vi "读取二维数组并转换到簇_new.vi"() -> (11 "Port 0":T1)   [LabVIEW 2021]
uses:
  <vilib>/Utility/file.llb/Read Delimited Spreadsheet (DBL).vi
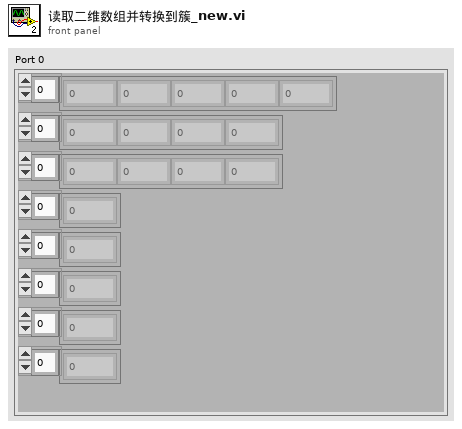
[diagram p1: front panel]
types:
  T1 = cluster{dbl[], dbl[], dbl[], dbl[], dbl[], dbl[], dbl[], dbl[]}
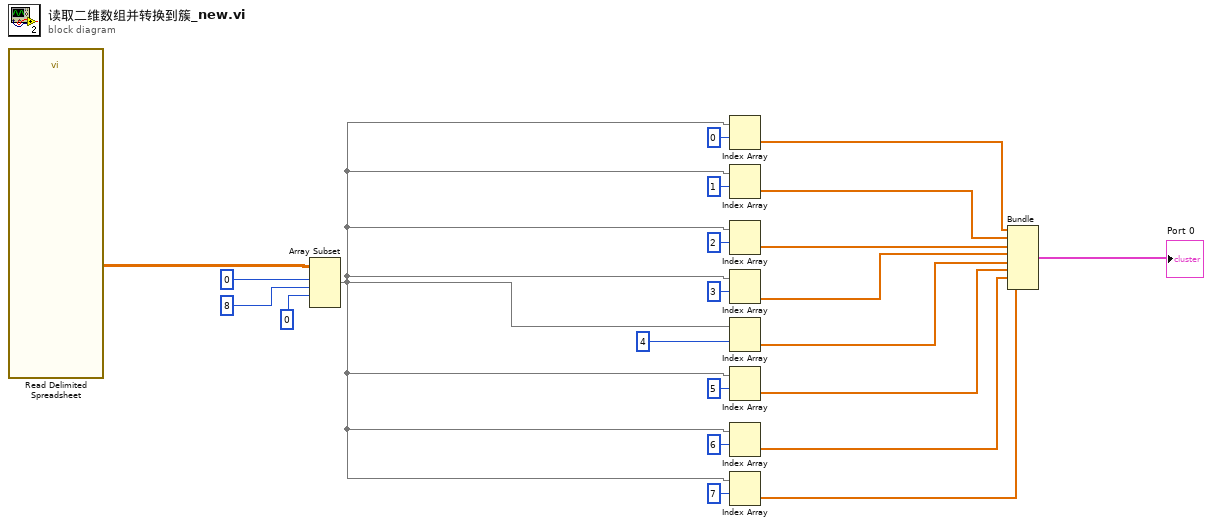
[diagram p0: block diagram]
diagram:
  n1 = call-poly <vilib>:"Read Delimited Spreadsheet.vi"() -> ("all rows"=w1:dbl[][])  [unwired: 10 in, 5 out]
  n2 = Array Subset(array=w1, index (row)=0 ("index"), length (row)=8 ("length"), index (col)=0 ("index")) -> (w12:dbl[][])  [unwired: 1 in]
  n3 = Index Array(array=w12, index (row)=0) -> (element=w11:dbl[])  [unwired: 1 in]
  n4 = Index Array(array=w12, index (row)=1) -> (element=w10:dbl[])  [unwired: 1 in]
  n5 = Index Array(array=w12, index (row)=2) -> (element=w9:dbl[])  [unwired: 1 in]
  n6 = Index Array(array=w12, index (row)=3) -> (element=w8:dbl[])  [unwired: 1 in]
  n7 = Index Array(array=w12, index (row)=4) -> (element=w3:dbl[])  [unwired: 1 in]
  n8 = Index Array(array=w12, index (row)=5) -> (element=w7:dbl[])  [unwired: 1 in]
  n9 = Index Array(array=w12, index (row)=6) -> (element=w6:dbl[])  [unwired: 1 in]
  n10 = Index Array(array=w12, index (row)=7) -> (element=w5:dbl[])  [unwired: 1 in]
  n11 = Bundle(w11, w10, w9, w8, w3, w7, w6, w5) -> (→"Port 0":T1)  [unwired: 1 in]
